vi "tap_stimulus_advanced.vi"(2 "Input Array":dbl[](array[numeric]), 3 "Cluster":T1) -> (0 "Timing array changed?":bool, 1 "Output Array":dbl[](array[numeric]))   [LabVIEW 2010]
panel:
  in  "Tap Train Number":i32[][](array[numeric])
  in  "Time between tap onset (ms)":i32[][](array[numeric])=[[0, 10]] min=3 max=6500
  in  "Duty Cycle":dbl[][](array[numeric])=[[0.0, 0.6]]
  out "tap number range":string
  out "tap interval range":string
  out "duty cycle range":string
  in  "stop":bool
  in  "OK Button":bool
  in  "Tap Stimulus Timing Array":dbl[](array[numeric])
  # "Tap Stimulus Timing Array (ms)"
  # "Duty Cycle"
  # "Switch time (ms)"
  # "Time between tap onset (ms)"
  # "Switch time (ms)"
  # "Tap Train Number"
  # "Switch time (ms)"
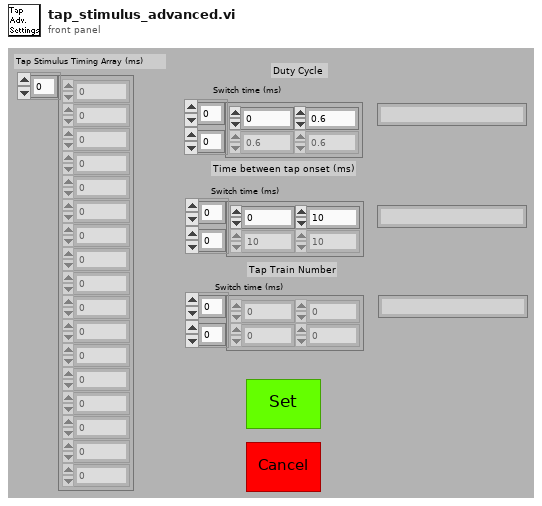
[diagram p1: front panel]
types:
  T1 = cluster{"tap fraction of time between is active":refnum<vi>, "time between tap onset":refnum<vi>, "Tap Train Number":refnum<vi>}
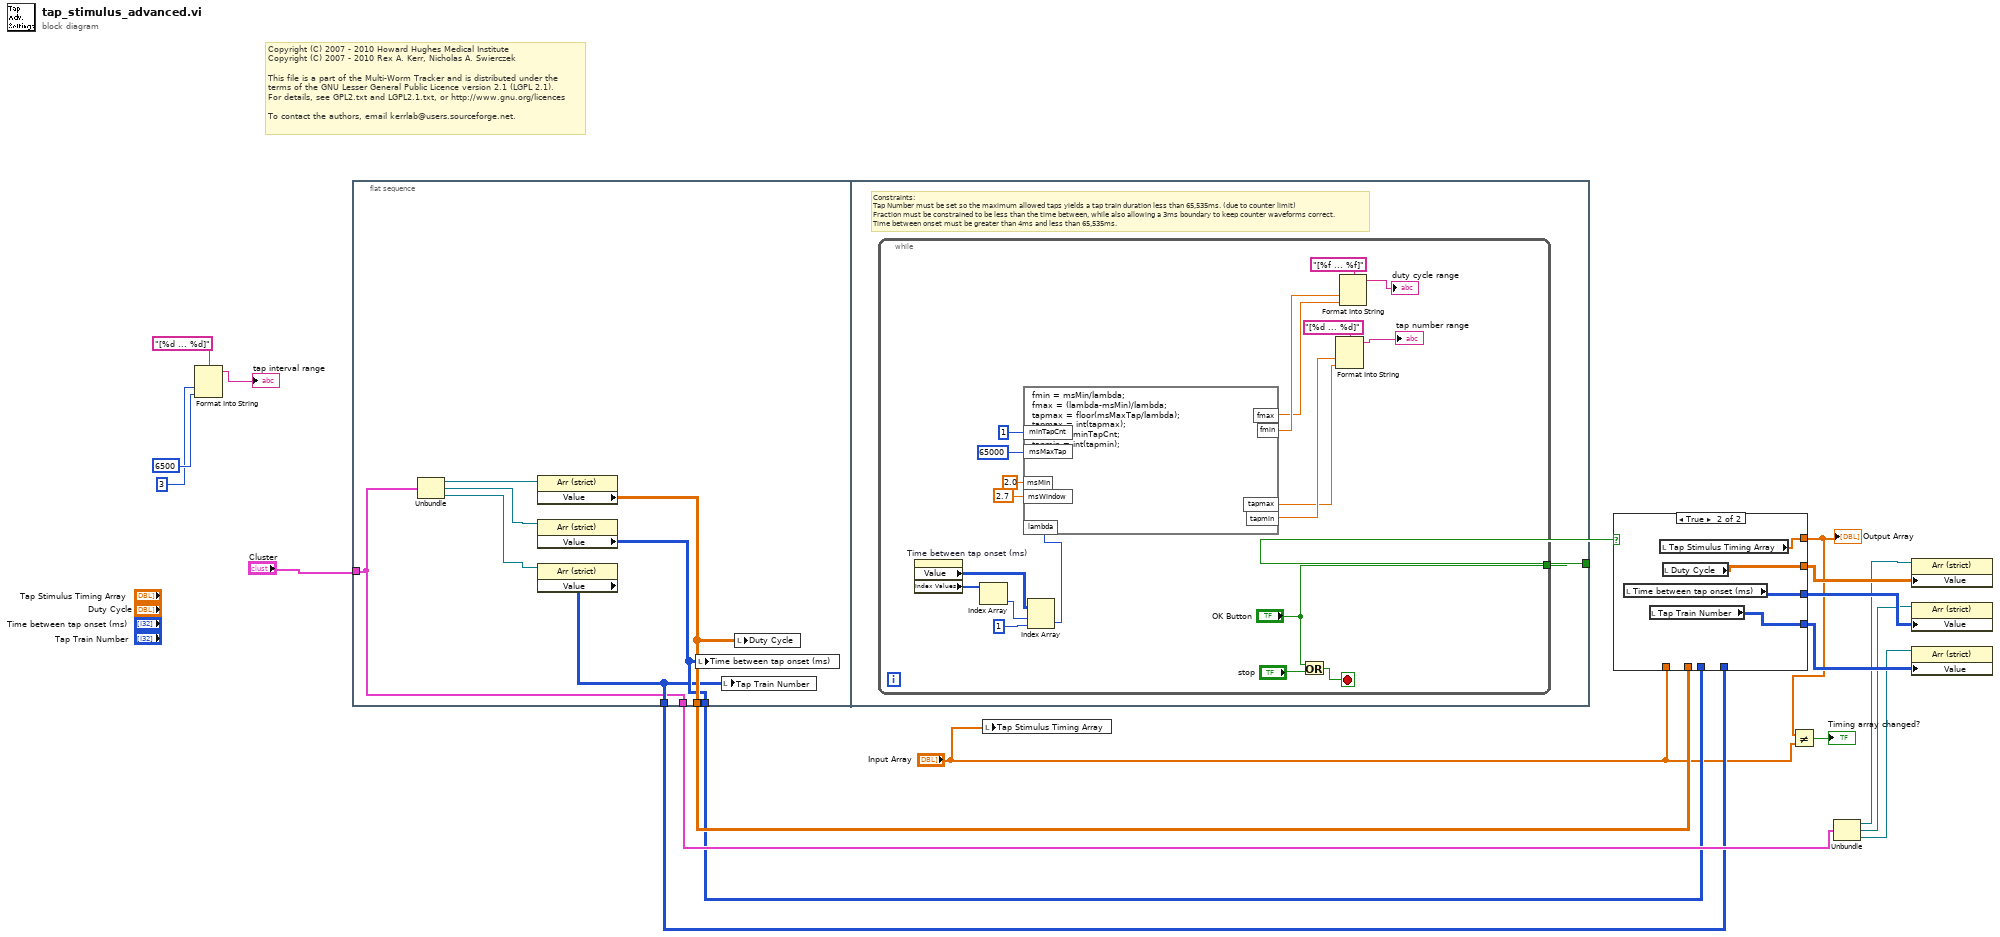
[diagram p0: block diagram]
diagram:
  # "Copyright (C) 2007 - 2010 Howard Hughes Medical Institute\nCopyright (C) 2007 - 2010 Rex A. Kerr, Nicholas A. Swierczek\n \nThis file is a part of the Multi-Worm Tracker and is distributed under the\nterms of the GNU Lesser General Public Licence version 2.1 (LGPL 2.1).\nFor details, see GPL2.txt and LGPL2.1.txt, or http://www.gnu.org/licences\n \nTo contact the authors, email kerrlab@users.sourceforge.net."
  n1 = Format Into String(format string="[%d ... %d]", 3 ("Data Entry Limits:Minimum"), 6500 ("x")) -> (resulting string=→"tap interval range":string)  [unwired: 2 in, 1 out]
  n2 = flat-sequence {
    tunnel: [w20] -> w10
    tunnel: [w23] -> w9
    tunnel: [w22] -> w8
    tunnel: [w21] -> w7
    tunnel: "Cluster" -> [w20]
    tunnel: [w27] -> w16
    frame #0 {
      n3 = Unbundle(w20) -> ("tap fraction of time between is active"=w24:refnum<vi>, "time between tap onset"=w25:refnum<vi>, "Tap Train Number"=w26:refnum<vi>)
      n4 = property class="Arr (strict)"(reference=w24) -> ("Value"=w23:sgl[][])  [unwired: 1 in, 2 out]
      n5 = property class="Arr (strict)"(reference=w25) -> ("Value"=w22:i32[][])  [unwired: 1 in, 2 out]
      n6 = property class="Arr (strict)"(reference=w26) -> ("Value"=w21:i32[][])  [unwired: 1 in, 2 out]
      n7 = local write "Time between tap onset (ms)"(w22) -> ()
      n8 = local write "Tap Train Number"(w21) -> ()
      n9 = local write "Duty Cycle"(w23) -> ()
    }
    frame #1 {
      # "Constraints:\nTap Number must be set so the maximum allowed taps yields a tap train duration less than 65,535ms. (due to counter limit)\nFraction must be constrained to be less than the time between, while also allowing a 3ms boundary to keep counter waveforms correct.\nTime between onset must be greater than 4ms and less than 65,535ms."
      n10 = while {
        tunnel: ["OK Button"] -> w27
        stop <- w47 stop-if-true
        n11 = property on="Time between tap onset (ms)" class="Arr (strict)"() -> ("Value"=w32:i32[][], "Index Values"=w29:u32[])  [unwired: 2 in, 2 out]
        n12 = Index Array(array=w29) -> (element=w28:u32)  [unwired: 1 in]
        n13 = Index Array(array=w32, index (row)=w28, index (col)=1 ("disabled index (col)")) -> (element=w31:i32)
        n14 = formula code="fmin = msMin/lambda;\nfmax = (lambda-msMin)/lambda;\ntapmax = floor(msMaxTap/lambda);\ntapmax = int(tapmax);\ntapmin = minTapCnt;\ntapmin = int(tapmin);"("minTapCnt"=1 ("input variable"), "msMaxTap"=65000 ("input variable"), "msMin"=2.0 ("input variable"), "lambda"=w31, "msWindow"=2.7 ("input variable")) -> ("fmin"=w39:dbl, "fmax"=w38:dbl, "tapmin"=w35:dbl, "tapmax"=w33:dbl)
        n15 = Or(x="OK Button", y="stop") -> (x .or. y?=w47:bool)
        n16 = Format Into String(format string="[%d ... %d]", w35, w33) -> (resulting string=→"tap number range":string)  [unwired: 2 in, 1 out]
        n17 = Format Into String(format string="[%f ... %f]", w39, w38) -> (resulting string=→"duty cycle range":string)  [unwired: 2 in, 1 out]
      }
    }
  }
  n18 = local write "Tap Stimulus Timing Array"("Input Array") -> ()
  n19 = case shown="True" w16 {
    tunnel: "Input Array" -> [w51 _]
    tunnel: [w51 w55] -> w2
    tunnel: [w50 w54] -> w19
    tunnel: [w49 w53] -> w18
    tunnel: [w48 w52] -> w17
    tunnel: w9 -> [w50 _]
    tunnel: w8 -> [w49 _]
    tunnel: w7 -> [w48 _]
    frame False {
    }
    frame True {
      n20 = local read "Time between tap onset (ms)"() -> (w53:i32[][])
      n21 = local read "Tap Train Number"() -> (w52:i32[][])
      n22 = local read "Tap Stimulus Timing Array"() -> (w55:dbl[])
      n23 = local read "Duty Cycle"() -> (w54:dbl[][])
    }
  }
  "Output Array" <- w2
  n24 = Not Equal?(x=w2, y="Input Array") -> (x != y?=→"Timing array changed?":bool)
  n25 = Unbundle(w10) -> ("tap fraction of time between is active"=w15:refnum<vi>, "time between tap onset"=w14:refnum<vi>, "Tap Train Number"=w13:refnum<vi>)
  n26 = property class="Arr (strict)"(reference=w15, "Value"=w19) -> ()  [unwired: 1 in, 2 out]
  n27 = property class="Arr (strict)"(reference=w14, "Value"=w18) -> ()  [unwired: 1 in, 2 out]
  n28 = property class="Arr (strict)"(reference=w13, "Value"=w17) -> ()  [unwired: 1 in, 2 out]
